vi "LiCor_setting_manager.vi"(1 "string to write":string="(RS232(Poll Now))", 2 "LiCor session in":T1={"VISA resource out"="COM12", "error out"={"status"=FALSE, "code"=0, "source"=""}}) -> (0 "LiCor session out":T1={"VISA resource out"="COM12", "error out"={"status"=FALSE, "code"=0, "source"=""}})   [LabVIEW 2010]
panel:
  # "This VI is for managing LiCor settings.\n\nThere is no need to enter carriage returns or line feeds (command termination characters) in the \"string to write\" input. This should be taken care of as long as this VI follows the LiCor_init VI in your custom VI flow."
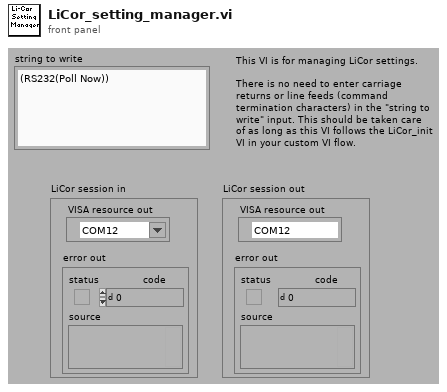
[diagram p1: front panel]
types:
  T1 = cluster{"VISA resource out":refnum<visa-resource-name>, "error out":errorcluster}
  T2 = cluster{"VISA session out":refnum<visa-resource-name>, "error out":errorcluster}
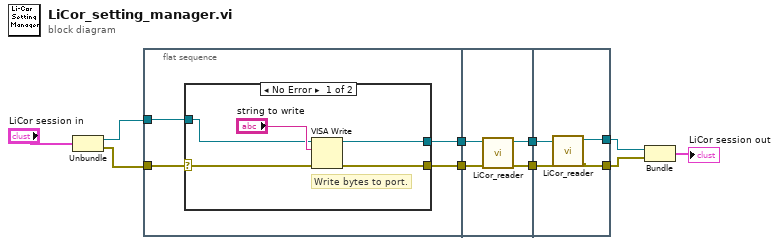
[diagram p0: block diagram]
diagram:
  n1 = Unbundle("LiCor session in") -> ("VISA resource out"=w5:refnum<visa-resource-name>, "error out"=w4:errorcluster)
  n2 = flat-sequence {
    tunnel: w5 -> [w14]
    tunnel: w4 -> [w13]
    tunnel: [w12] -> w10
    tunnel: [w11] -> w9
    tunnel: w10 -> [w25]
    tunnel: w9 -> [w24]
    tunnel: [w23] -> w8
    tunnel: [w22] -> w7
    tunnel: w8 -> [w29]
    tunnel: w7 -> [w28]
    tunnel: [w27] -> w3
    tunnel: [w26] -> w2
    frame #0 {
      n3 = case shown="No Error" w13 {
        selector: w13 -> [w15 w21]
        tunnel: [w19 w20] -> w12
        tunnel: [w18 w21] -> w11
        tunnel: w14 -> [w16 w20]
        frame No Error {
          # "Write bytes to port."
          n4 = VISA Write(VISA resource name=w16, write buffer="string to write", error in (no error)=w15) -> (VISA resource name out=w19:refnum<visa-resource-name>, error out=w18:errorcluster)  [unwired: 1 out]
        }
        frame Error {
        }
      }
    }
    frame #1 {
      n5 = call "LiCor_reader.vi"("error in"=w24, "VISA session in"=w25) -> ("error out"=w22:errorcluster, "VISA session out"=w23:refnum<visa-resource-name>)  [unwired: 6 in, 2 out]
    }
    frame #2 {
      n6 = call "LiCor_reader.vi"("error in"=w28, "VISA session in"=w29) -> ("error out"=w26:errorcluster, "VISA session out"=w27:refnum<visa-resource-name>)  [unwired: 6 in, 2 out]
    }
  }
  n7 = Bundle("VISA session out"=w3, "error out"=w2) -> (→"LiCor session out":T2)  [unwired: 1 in]
